vi "connect.vi"(8 "error in (no error)":errorcluster, 11 "OHAUS_232 in":refnum<class "OHAUS_Navigator_232.lvclass">) -> (0 "error out":errorcluster, 3 "OHAUS_232 out":refnum<class "OHAUS_Navigator_232.lvclass">)   [LabVIEW 2019, in "OHAUS_Navigator_232.lvclass"]
uses:
  OHAUS_Navigator_232.lvclass
  OHAUS_Navigator_232.lvclass/OHAUS_Navigator_232.ctl
  <vilib>/Instr/_visa.llb/VISA Configure Serial Port (Instr).vi
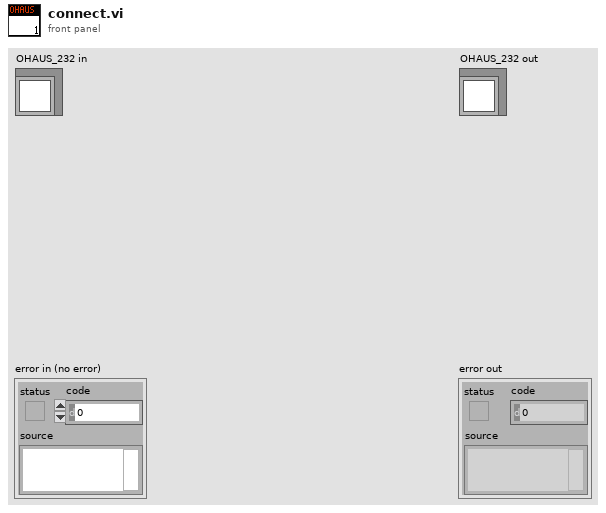
[diagram p1: front panel]
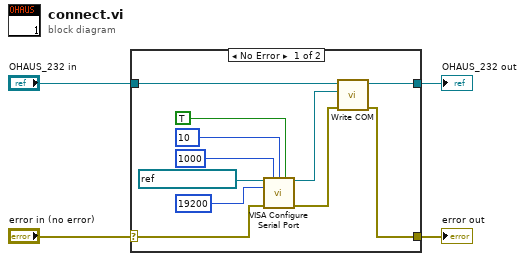
[diagram p0: block diagram]
diagram:
  n1 = case shown="No Error" "error in (no error)" {
    selector: "error in (no error)" -> [w10 w17]
    tunnel: [w5 w17] -> w3
    tunnel: [w9 w16] -> w1
    tunnel: "OHAUS_232 in" -> [w8 w16]
    frame No Error {
      n2 = call-poly "VISA Configure Serial Port"("VISA resource name"=refnum<visa-resource-name> "ASRL1::INSTR", "timeout (10sec)"=u32 1000, "termination char\n(0xA = '\\n' = LF)"=u8 10 ("termination char\n(0xA = '\\n' = LF)"), "Enable Termination\nChar (T)"=TRUE ("Enable Termination\nChar (T)"), "baud rate (9600)"=u32 19200, "error in (no error)"=w10) -> ("VISA resource name out"=w6:refnum<visa-resource-name>, "error out"=w7:errorcluster)  [unwired: 8 in]
      n3 = call "Write COM.vi"("error in (no error)"=w7, "COM"=w6, "OHAUS_Navigator_232 in"=w8) -> ("error out"=w5:errorcluster, "OHAUS_Navigator_232 out"=w9:refnum<class "OHAUS_Navigator_232.lvclass">)  [unwired: 7 in]
    }
    frame Error {
    }
  }
  "error out" <- w3
  "OHAUS_232 out" <- w1
